vi "save channels to interleaved tiff series.vi"(8 "frame number in":i32, 9 "last frame":bool, 11 "image data in":dbl[][](array[numeric])) -> ()   [LabVIEW 2012]
uses:
  Custom Controls/file format type def.ctl
  GFG/GFGpathGet.vi
  GFG/GFGnumericGet.vi
  GFG/GFG library.lvlib
  Libtiff3/libtiff3.llb/libtiff3.lvlib
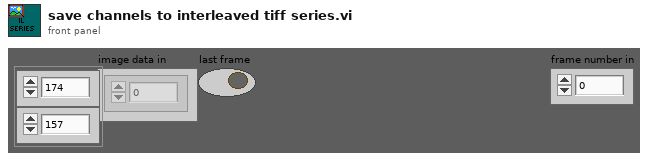
[diagram p1: front panel]
types:
  T1 = typedef "file format type def.ctl" = enum16{"16bit raw", "32bit raw", "16bit multi-tiff (interleave)", "16bit multi-tiff (separate)", "16bit multi-tiff (stacked)", "32bit multi-tiff (interleave)", "32bit multi-tiff (separate)", "32bit multi-tiff (stacked)", "16bit tiff series (interleave)", "16bit tiff series (separate)", "16bit tiff series (stacked)", "32bit tiff series (interleave)", "32bit tiff series (separate)", "32bit tiff series (stacked)"}
  T2 = cluster{"no..of.frames.to.acquire":dbl, "x.pixels":dbl, "y.pixels":dbl, "x.pixel.sz":dbl, "y.pixel.sz":dbl}
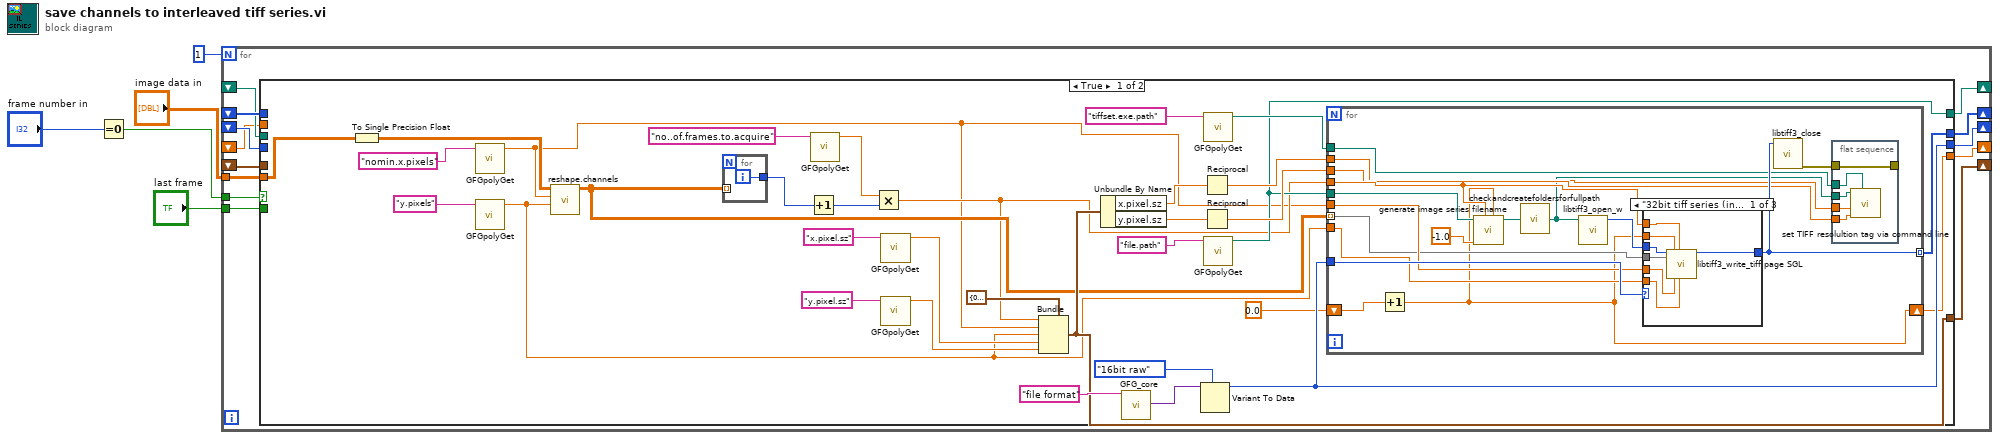
[diagram p0: block diagram]
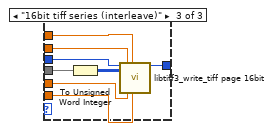
[diagram p3: hidden frame]
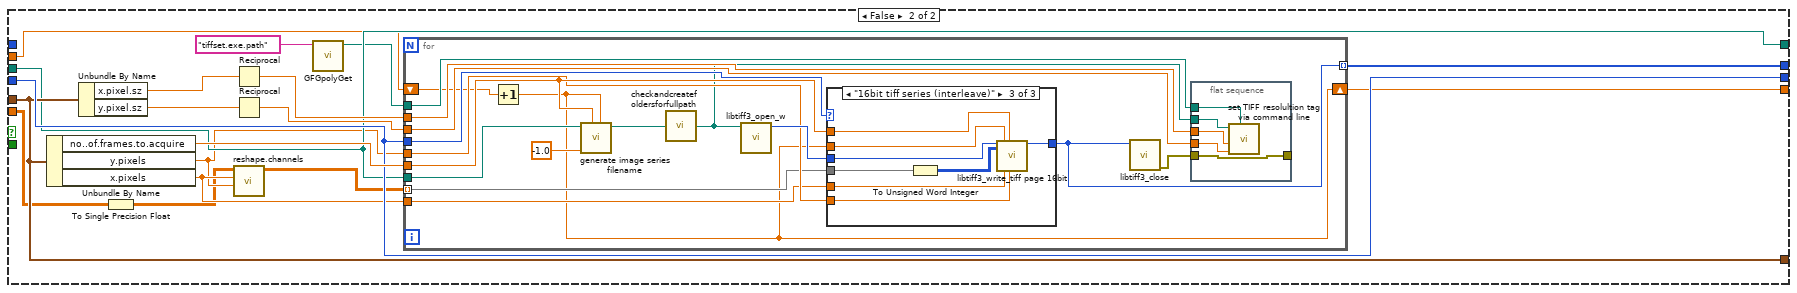
[diagram p4: hidden frame]
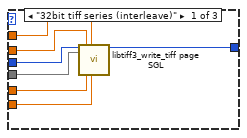
[diagram p5: hidden frame]
diagram:
  n1 = Equal To 0?(x="frame number in") -> (x = 0?=w4:bool)
  n2 = for {
    N: 1 -> [_]
    tunnel: w4 -> [w18]
    shift-right: [w17] -> _
    shift-left: _ -> [w16]
    tunnel: "image data in" -> [w15]
    shift-right: [w14] -> _
    shift-left: _ -> [w13]
    shift-right: [w12] -> _
    shift-left: _ -> [w11]
    shift-right: [w10] -> _
    shift-left: _ -> [w9]
    tunnel: "last frame" -> [w8]
    shift-right: [w7] -> _
    shift-left: _ -> [w6]
    n3 = case shown="True" w18 {
      tunnel: w13 -> [_ w107]
      tunnel: [w38 w105] -> w17
      tunnel: w16 -> [_ _]
      tunnel: w15 -> [w28 w96]
      tunnel: [w39 w107] -> w14
      tunnel: [w37 w106] -> w12
      tunnel: w11 -> [_ w106]
      tunnel: [w30 w99] -> w10
      tunnel: w9 -> [_ w99]
      tunnel: w8 -> [_ _]
      tunnel: [w25 w91] -> w7
      tunnel: w6 -> [_ w92]
      frame True {
        n4 = To Single Precision Float(number=w28) -> (single precision float=w29:sgl[][])
        n5 = call-poly "GFGpolyGet.vi"("Variable Name in"="nomin.x.pixels" ("Tag in")) -> ("Numeric"=w19:dbl)  [unwired: 9 in, 1 out]
        n6 = call-poly "GFGpolyGet.vi"("Variable Name in"="y.pixels" ("Tag in")) -> ("Numeric"=w27:dbl)  [unwired: 9 in, 1 out]
        n7 = call "reshape.channels.vi"("y.pixels"=w27, "x.pixels"=w19, "element"=w29) -> ("Array"=w24:dbl[][][])  [unwired: 8 in]
        n8 = for {
          tunnel: w24 -> [_] mode=indexing
          tunnel: [w52] -> w22
          i -> [w52]
        }
        n9 = Increment(x=w22) -> (x+1=w21:i32)
        n10 = call-poly "GFGpolyGet.vi"("Variable Name in"="no..of.frames.to.acquire") -> ("Numeric"=w23:dbl)  [unwired: 9 in, 1 out]
        n11 = Multiply(x=w23, y=w21) -> (x*y=w20:dbl)
        n12 = call-poly "GFGpolyGet.vi"("Variable Name in"="x.pixel.sz" ("Tag in")) -> ("Numeric"=w42:dbl)  [unwired: 9 in, 1 out]
        n13 = call-poly "GFGpolyGet.vi"("Variable Name in"="y.pixel.sz" ("Tag in")) -> ("Numeric"=w41:dbl)  [unwired: 9 in, 1 out]
        n14 = Bundle(cluster=T2 {"no..of.frames.to.acquire"=0.0, "x.pixels"=0.0, "y.pixels"=0.0, "x.pixel.sz"=0.0, "y.pixel.sz"=0.0} ("output cluster"), "no..of.frames.to.acquire"=w20, "x.pixels"=w19, "y.pixels"=w27, "x.pixel.sz"=w42, "y.pixel.sz"=w41) -> (w37:T2)
        n15 = Unbundle By Name(w37) -> ("x.pixel.sz"=w33:dbl, "y.pixel.sz"=w34:dbl)
        n16 = call "GFG_core.vi"("Variable Name in"="file format") -> ("Variant Out"=w50:variant)  [unwired: 12 in, 6 out]
        n17 = Variant To Data(type=file_format_type_def."16bit raw" ("file format"), Variant=w50) -> (data=w39:T1)  [unwired: 1 in, 1 out]
        n18 = Reciprocal(x=w33) -> (1/x=w35:dbl)
        n19 = Reciprocal(x=w34) -> (1/x=w36:dbl)
        n20 = call-poly "GFGpolyGet.vi"("Variable Name in"="tiffset.exe.path") -> ("Path"=w31:path)  [unwired: 9 in, 1 out]
        n21 = call-poly "GFGpolyGet.vi"("Variable Name in"="file.path") -> ("Path"=w30:path)  [unwired: 9 in, 1 out]
        n22 = for {
          tunnel: w39 -> [w69]
          tunnel: w19 -> [w67]
          tunnel: w27 -> [w66]
          tunnel: w20 -> [w64]
          tunnel: [w63] -> w38 mode=indexing
          tunnel: w36 -> [w61]
          tunnel: w35 -> [w60]
          tunnel: w31 -> [w59]
          tunnel: w30 -> [w58]
          tunnel: w24 -> [w57] mode=indexing
          shift-right: [w53] -> w25
          shift-left: 0.0 -> [w55]
          n23 = Increment(x=w55) -> (x+1=w53:dbl)
          n24 = call "generate image series filename.vi"("frame number in"=w53, "no..of.frames.to.acquire"=w64, "channel"=-1.0, "Path IN"=w58) -> ("appended path"=w65:path)  [unwired: 7 in]
          n25 = call "checkandcreatefoldersforfullpath.vi"("Path IN"=w65) -> ("Path OUT"=w56:path)  [unwired: 4 in]
          n26 = call "libtiff3_open_w.vi"("Input path"=w56) -> ("handle"=w68:i32)  [unwired: 9 in, 1 out]
          n27 = case shown="\"32bit tiff series (interleave)\"" w69 {
            tunnel: w57 -> [w75 _ w87]
            tunnel: w68 -> [w78 w82 w88]
            tunnel: w53 -> [w79 _ w89]
            tunnel: w64 -> [w80 _ w90]
            tunnel: [w81 w82 w83] -> w63
            tunnel: w67 -> [w76 _ w85]
            tunnel: w66 -> [w77 _ w84]
            frame "32bit tiff series (interleave)" {
              n28 = call "libtiff3_write_tiff page SGL.vi"("Handle"=w78, "Image Pixels (Float)"=w75, "page"=w79, "x.pixels"=w76, "totalpages"=w80, "y.pixels"=w77) -> ("Handle out"=w81:i32)  [unwired: 12 in, 1 out]
            }
            frame Default {
            }
            frame "16bit tiff series (interleave)" {
              n29 = To Unsigned Word Integer(number=w87) -> (unsigned 16bit integer=w86:u16[][])
              n30 = call "libtiff3_write_tiff page 16bit.vi"("Handle"=w88, "Image Pixels (U16)"=w86, "page"=w89, "x.pixels"=w85, "totalpages"=w90, "y.pixels"=w84) -> ("Handle out"=w83:i32)  [unwired: 12 in, 1 out]
            }
          }
          n31 = call "libtiff3_close.vi"("Handle"=w63) -> ("error out"=w62:errorcluster)  [unwired: 9 in]
          n32 = flat-sequence {
            tunnel: w62 -> [w72]
            tunnel: w60 -> [w74]
            tunnel: w61 -> [w73]
            tunnel: [w72] -> _
            tunnel: w59 -> [w71]
            tunnel: w56 -> [w70]
            frame #0 {
              n33 = call "set TIFF resolultion tag via command line.vi"("tiffset.exe file path"=w71, "y pixels per m"=w73, "x pixels per m"=w74, "TIFF file path"=w70) -> ()  [unwired: 8 in]
            }
          }
        }
      }
      frame False {
        n34 = Unbundle By Name(w106) -> ("no..of.frames.to.acquire"=w108:dbl, "y.pixels"=w97:dbl, "x.pixels"=w98:dbl)
        n35 = Unbundle By Name(w106) -> ("x.pixel.sz"=w101:dbl, "y.pixel.sz"=w102:dbl)
        n36 = To Single Precision Float(number=w96) -> (single precision float=w95:sgl[][])
        n37 = Reciprocal(x=w101) -> (1/x=w103:dbl)
        n38 = Reciprocal(x=w102) -> (1/x=w104:dbl)
        n39 = call "reshape.channels.vi"("y.pixels"=w97, "x.pixels"=w98, "element"=w95) -> ("Array"=w94:dbl[][][])  [unwired: 8 in]
        n40 = call-poly "GFGpolyGet.vi"("Variable Name in"="tiffset.exe.path") -> ("Path"=w93:path)  [unwired: 9 in, 1 out]
        n41 = for {
          tunnel: w108 -> [w123]
          tunnel: w107 -> [w122]
          tunnel: w97 -> [w121]
          tunnel: w98 -> [w120]
          tunnel: [w119] -> w105 mode=indexing
          tunnel: w104 -> [w117]
          tunnel: w103 -> [w116]
          tunnel: w99 -> [w115]
          tunnel: w94 -> [w114] mode=indexing
          tunnel: w93 -> [w113]
          shift-right: [w109] -> w91
          shift-left: w92 -> [w111]
          n42 = Increment(x=w111) -> (x+1=w109:dbl)
          n43 = call "generate image series filename.vi"("frame number in"=w109, "no..of.frames.to.acquire"=w123, "channel"=-1.0, "Path IN"=w115) -> ("appended path"=w124:path)  [unwired: 7 in]
          n44 = call "checkandcreatefoldersforfullpath.vi"("Path IN"=w124) -> ("Path OUT"=w112:path)  [unwired: 4 in]
          n45 = call "libtiff3_open_w.vi"("Input path"=w112) -> ("handle"=w125:i32)  [unwired: 9 in, 1 out]
          n46 = case shown="\"16bit tiff series (interleave)\"" w122 {
            tunnel: w114 -> [w131 _ w143]
            tunnel: w125 -> [w134 w138 w144]
            tunnel: w109 -> [w135 _ w145]
            tunnel: w123 -> [w136 _ w146]
            tunnel: [w137 w138 w139] -> w119
            tunnel: w120 -> [w132 _ w141]
            tunnel: w121 -> [w133 _ w140]
            frame "32bit tiff series (interleave)" {
              n47 = call "libtiff3_write_tiff page SGL.vi"("Handle"=w134, "Image Pixels (Float)"=w131, "page"=w135, "x.pixels"=w132, "totalpages"=w136, "y.pixels"=w133) -> ("Handle out"=w137:i32)  [unwired: 12 in, 1 out]
            }
            frame Default {
            }
            frame "16bit tiff series (interleave)" {
              n48 = To Unsigned Word Integer(number=w143) -> (unsigned 16bit integer=w142:u16[][])
              n49 = call "libtiff3_write_tiff page 16bit.vi"("Handle"=w144, "Image Pixels (U16)"=w142, "page"=w145, "x.pixels"=w141, "totalpages"=w146, "y.pixels"=w140) -> ("Handle out"=w139:i32)  [unwired: 12 in, 1 out]
            }
          }
          n50 = call "libtiff3_close.vi"("Handle"=w119) -> ("error out"=w118:errorcluster)  [unwired: 9 in]
          n51 = flat-sequence {
            tunnel: w118 -> [w128]
            tunnel: w116 -> [w130]
            tunnel: w117 -> [w129]
            tunnel: [w128] -> _
            tunnel: w113 -> [w127]
            tunnel: w112 -> [w126]
            frame #0 {
              n52 = call "set TIFF resolultion tag via command line.vi"("tiffset.exe file path"=w127, "y pixels per m"=w129, "x pixels per m"=w130, "TIFF file path"=w126) -> ()  [unwired: 8 in]
            }
          }
        }
      }
    }
  }
